vi "Hi-Tec_calibs.vi"(5 "Gas Line Name":string) -> (1 "Hi-Tec calib":T1={"Ref temp (deg C)"=0.0, "Ref Pres (mbars)"=0.0, "Density at calib conditions"=-0.0141, "Coefficients"=[]} {"Coefficients" format="%.2f"; "Density at calib conditions" format="%.4f"; "Ref Pres (mbars)" format="%.2f"; "Ref temp (deg C)" format="%.2f"}, 2 "Comments":string)   [LabVIEW 2010]
uses:
  Controls/Hi-Tec_calib.ctl
  Anemometry/Anemometry Sub Vis/Globals/Gas_management_global.vi
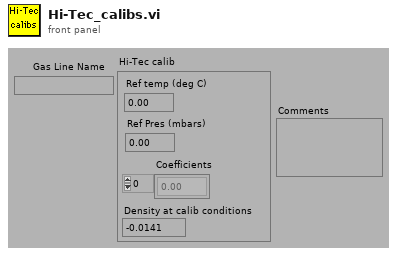
[diagram p1: front panel]
types:
  T1 = typedef "Hi-Tec_calib.ctl" = cluster{"Ref temp (deg C)":dbl, "Ref Pres (mbars)":dbl, "Density at calib conditions":dbl, "Coefficients":dbl[]}
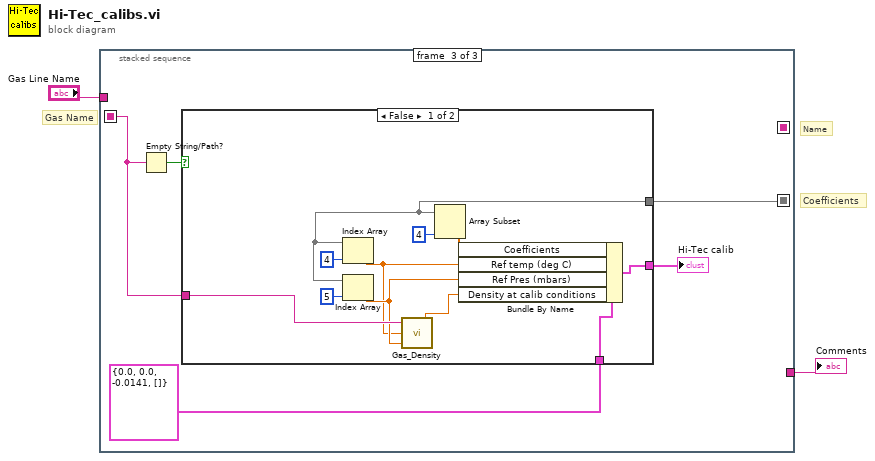
[diagram p0: block diagram]
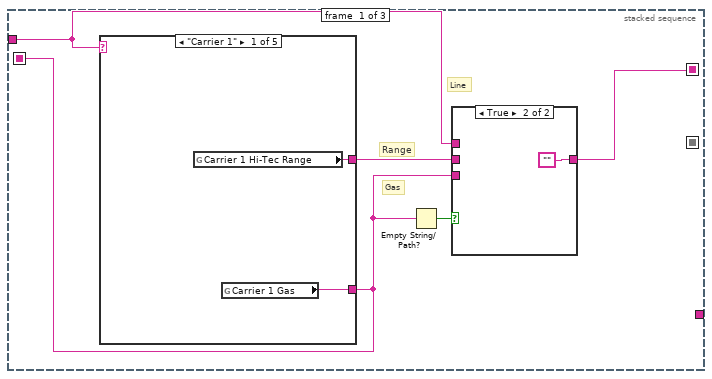
[diagram p2: hidden frame]
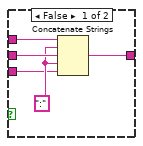
[diagram p3: hidden frame]
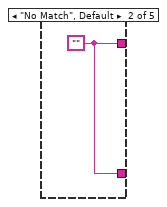
[diagram p4: hidden frame]
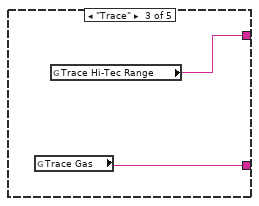
[diagram p5: hidden frame]
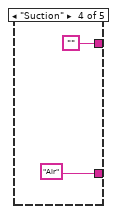
[diagram p6: hidden frame]
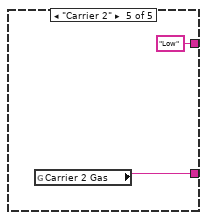
[diagram p7: hidden frame]
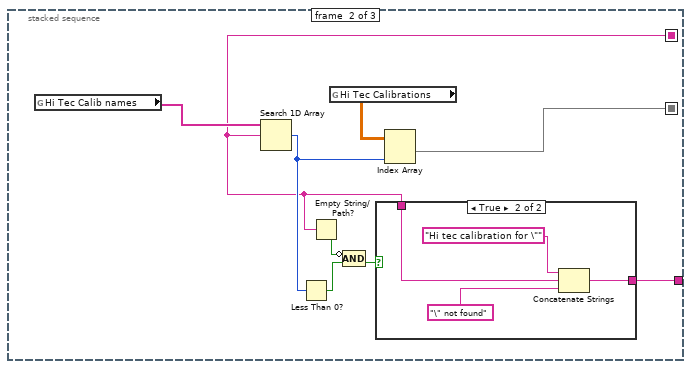
[diagram p8: hidden frame]
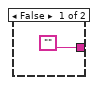
[diagram p9: hidden frame]
diagram:
  # "Name"
  # "Coefficients"
  # "Gas Name"
  n1 = stacked-sequence {
    seq-local: [w5 _ _] -> [_ _ w40]
    seq-local: [_ w29 _] -> [_ _ w37]
    seq-local: [w3 _ _] -> [_ w26 _]
    tunnel: "Gas Line Name" -> [w7 _ _]
    tunnel: [_ w27 _] -> w1
    frame #0 {
      # "Gas"
      # "Range"
      # "Line"
      n2 = case shown="\"Carrier 1\"" w7 {
        tunnel: [w14 w16 w18 "" "Low"] -> w6
        tunnel: [w15 w16 w17 "Air" ("Carrier 2 Gas") w22] -> w5
        frame "Carrier 1" {
          n3 = global read "Gas_management_global.vi" "Carrier 1 Hi-Tec Range"() -> (w14:string)
          n4 = global read "Gas_management_global.vi" "Carrier 1 Gas"() -> (w15:string)
        }
        frame "No Match", Default {
          w16 = ""
        }
        frame "Trace" {
          n5 = global read "Gas_management_global.vi" "Trace Gas"() -> (w17:string)
          n6 = global read "Gas_management_global.vi" "Trace Hi-Tec Range"() -> (w18:string)
        }
        frame "Suction" {
        }
        frame "Carrier 2" {
          n7 = global read "Gas_management_global.vi" "Carrier 2 Gas"() -> (w22:string)
        }
      }
      n8 = Empty String/Path?(string/path=w5) -> (empty?=w4:bool)
      n9 = case shown="True" w4 {
        tunnel: w7 -> [w12 _]
        tunnel: w6 -> [w11 _]
        tunnel: w5 -> [w9 _]
        tunnel: [w8 ""] -> w3
        frame False {
          w10 = ":"
          n10 = Concatenate Strings(w12, w10, w11, w10, w9) -> (w8:string)
        }
        frame True {
        }
      }
    }
    frame #1 {
      n11 = global read "Gas_management_global.vi" "Hi Tec Calib names"() -> (w31:string[])
      n12 = Search 1D Array(1D array=w31, element=w26) -> (index of element=w28:i32)  [unwired: 1 out]
      n13 = Less Than 0?(x=w28) -> (x < 0?=w24:bool)
      n14 = Empty String/Path?(string/path=w26) -> (empty?=w25:bool)
      n15 = global read "Gas_management_global.vi" "Hi Tec Calibrations"() -> (w30:dbl[][])
      n16 = Compound Arithmetic op=AND(invert w25, w24) -> (w23:bool)
      n17 = case shown="True" w23 {
        tunnel: w26 -> [_ w35]
        tunnel: ["" w33] -> w27
        frame False {
        }
        frame True {
          n18 = Concatenate Strings("Hi tec calibration for \"", w35, "\" not found") -> (w33:string)
        }
      }
      n19 = Index Array(array=w30, index (col)=w28) -> (element=w29:dbl[])  [unwired: 1 in]
    }
    frame #2 {
      n20 = Empty String/Path?(string/path=w40) -> (empty?=w41:bool)
      n21 = case shown="False" w41 {
        tunnel: w40 -> [w51 _]
        tunnel: w37 -> [w44 _]
        tunnel: [w50 w53] -> w39
        tunnel: T1 {"Ref temp (deg C)"=0.0, "Ref Pres (mbars)"=0.0, "Density at calib conditions"=-0.0141, "Coefficients"=[]} ("Hi-Tec calib") -> [w49 w53]
        frame False {
          n22 = Index Array(array=w44, index=4) -> (element=w42:dbl)
          n23 = Index Array(array=w44, index=5) -> (element=w43:dbl)
          n24 = call "Gas_Density.vi"("Pressure (mbars)"=w43, "Temperature (deg C)"=w42, "Gas Name"=w51) -> ("Density Kg/m3"=w52:dbl)
          n25 = Array Subset(array=w44, length=4) -> (w47:dbl[])  [unwired: 1 in]
          n26 = Bundle By Name(cluster=w49, "Coefficients"=w47, "Ref temp (deg C)"=w42, "Ref Pres (mbars)"=w43, "Density at calib conditions"=w52) -> (w50:T1)
        }
        frame True {
        }
      }
      "Hi-Tec calib" <- w39
    }
  }
  "Comments" <- w1
